vi "process.vi"(8 "error in":errorcluster, 9 "result allocation":T1, 10 "parameters":T1, 11 "Temperature Chamber Model runtime in":refnum<class "Temperature Chamber Model runtime.lvclass">) -> (0 "error out":errorcluster, 1 "results":T1, 2 "parameter allocation":T1, 3 "Temperature Chamber Model runtime out":refnum<class "Temperature Chamber Model runtime.lvclass">)   [LabVIEW 2013, in "Temperature Chamber Model runtime.lvclass"]
doc: "Provides an interface for information processing by a module at runtime. While this interface performs no operations, a child should provide an override which may process data in any manner necessary."
uses:
  Temperature Chamber Model runtime.lvclass
  <vilib>/NI/Tag Bus/table/data table.ctl
  <vilib>/NI/Tag Bus/table/data table.lvlib
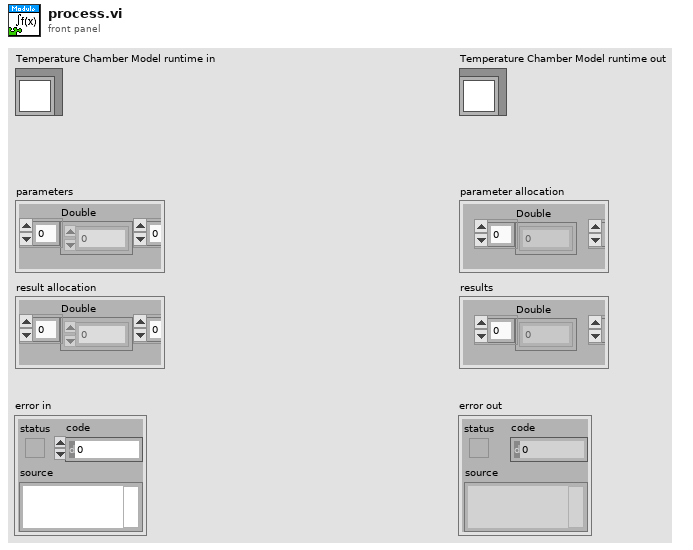
[diagram p1: front panel]
types:
  T1 = typedef "tag bus.lvlib/data table.lvlib/data table.ctl" = cluster{"Double":dbl[], "Single":sgl[], "I64":i64[], "I32":i32[], "I16":i16[], "I8":i8[], "U64":u64[], "U32":u32[], "U16":u16[], "U8":u8[], "Boolean":bool[], "String":string[], "Array of Double":cluster{"DBL Array":dbl[]}[], "Array of Single":cluster{"SGL Array":sgl[]}[], "Array of I64":cluster{"I64 Array":i64[]}[], "Array of I32":cluster{"I32 Array":i32[]}[], "Array of I16":cluster{"I16 Array":i16[]}[], "Array of I8":cluster{"I8 Array":i8[]}[], "Array of U64":cluster{"U64 Array":u64[]}[], "Array of U32":cluster{"U32 Array":u32[]}[], "Array of U16":cluster{"U16 Array":u16[]}[], "Array of U8":cluster{"U8 Array":u8[]}[], "Array of Boolean":cluster{"Boolean Array":bool[]}[], "Array of String":cluster{"String Array":string[]}[]}
  T2 = typedef "Temperature Chamber Model configuration.lvclass/parameter data indices.ctl" = cluster{"Double.Ambient Temperature":i32, "Double.Fan PWM":i32, "Double.Lamp PWM":i32}
  T3 = typedef "Temperature Chamber Model configuration.lvclass/result data indices.ctl" = cluster{"Double.Thermocouple Reading":i32}
  T4 = typedef "Temperature Chamber Model runtime.lvclass/model state.ctl" = cluster{"Previous Temperature":dbl, "Previous Tick Count":u32, "Just Initialized?":bool}
  T5 = typedef "Temperature Chamber Model runtime.lvclass/parameter user data.ctl" = cluster{"Ambient Temperature":dbl, "Fan PWM":dbl, "Lamp PWM":dbl}
  T6 = typedef "Temperature Chamber Model runtime.lvclass/result user data.ctl" = cluster{"Thermocouple Reading":dbl}
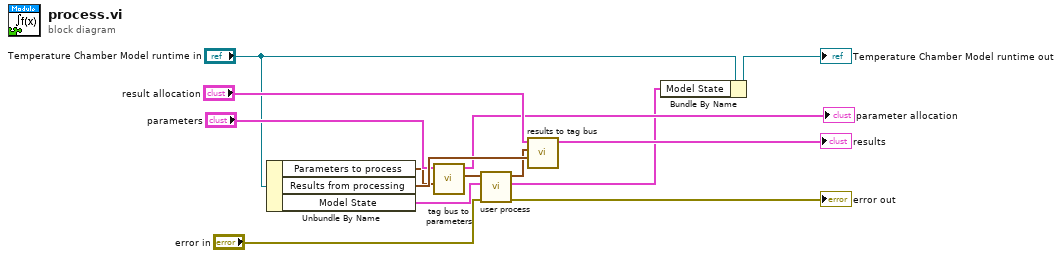
[diagram p0: block diagram]
diagram:
  n1 = Unbundle By Name("Temperature Chamber Model runtime in") -> ("Parameters to process"=w7:T2, "Results from processing"=w10:T3, "Model State"=w3:T4)
  n2 = call "tag bus to parameters.vi"("indices"=w7, "tag bus in"="parameters") -> ("data cluster"=w6:T5, "tag bus out"=→"parameter allocation":T1)  [unwired: 8 in]
  n3 = call "user process.vi"("error in"="error in", "Model State In"=w3, "Parameters to process"=w6) -> ("error out"=→"error out":errorcluster, "Model State Out"=w2:T4, "Results from processing"=w5:T6)  [unwired: 6 in]
  n4 = call "results to tag bus.vi"("indices"=w10, "data cluster"=w5, "tag bus in"="result allocation") -> ("tag bus out"=→"results":T1)  [unwired: 8 in]
  n5 = Bundle By Name(cluster="Temperature Chamber Model runtime in", "Model State"=w2) -> (→"Temperature Chamber Model runtime out":refnum<class "Temperature Chamber Model runtime.lvclass">)
